vi "Key.vi"(4 "Comment (Create only)":string, 6 "Operation (Read or Create)":T1, 7 "Section":string, 8 "error in (no error)":errorcluster, 9 "Value":string, 10 "Key":string, 11 "Ini Path in":path) -> (0 "error out":errorcluster, 1 "Found?":bool, 2 "Value out":string, 3 "Ini Path out":path)   [LabVIEW 2021, in "Config.lvlib"]
uses:
  Config.lvlib
  TypeDefs/Operation.ctl
  TypeDefs/Action.ctl
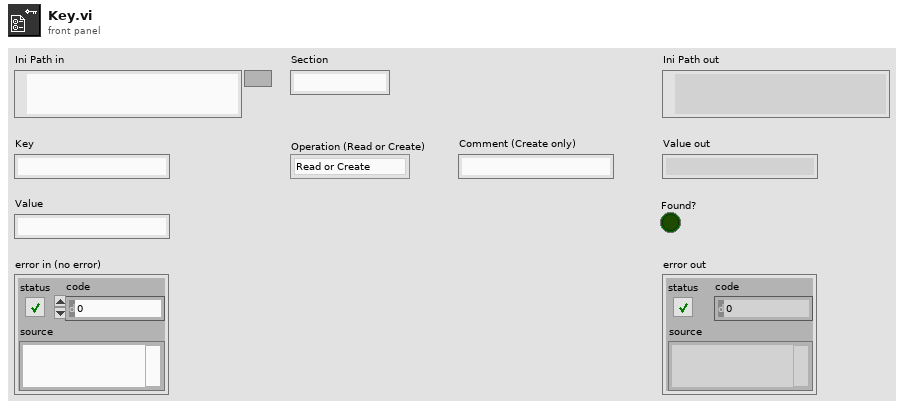
[diagram p1: front panel]
types:
  T1 = typedef "Config.lvlib/Operation.ctl" = enum8{"Read or Create", "Read", "Write"}
  T2 = typedef "Config.lvlib/Action.ctl" = enum8{"noop", "new", "read_or_create", "read", "write", "remove", "keys", "sections", "remove_section", "import", "export", "get", "set", "pop", "add", "list", "list_sections", "pop_section"}
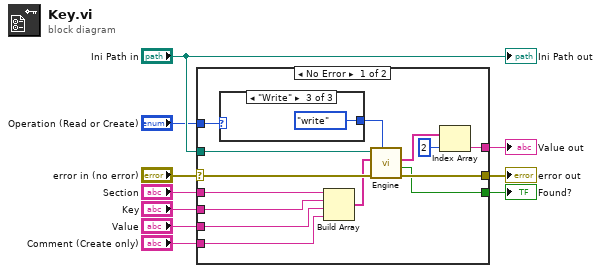
[diagram p0: block diagram]
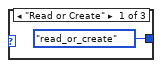
[diagram p2: hidden frame]
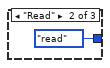
[diagram p3: hidden frame]
diagram:
  n1 = case shown="No Error" "error in (no error)" {
    selector: "error in (no error)" -> [w24 w29]
    tunnel: "Ini Path in" -> [w22 _]
    tunnel: [w21 w29] -> w8
    tunnel: "Section" -> [w20 _]
    tunnel: [w18 _] -> w6
    tunnel: "Key" -> [w17 _]
    tunnel: "Value" -> [w16 w28]
    tunnel: "Comment (Create only)" -> [w15 _]
    tunnel: "Operation (Read or Create)" -> [w14 _]
    tunnel: [w11 w28] -> w1
    frame No Error {
      n2 = case shown="\"Write\"" w14 {
        tunnel: [Action."read_or_create" ("Action") Action."read" ("Action") Action."write" ("Action")] -> w23
        frame "Read or Create" {
        }
        frame "Read" {
        }
        frame "Write" {
        }
      }
      n3 = Build Array(w20, w17, w16, w15) -> (w19:string[])
      n4 = call "Engine.vi"("Action"=w23, "error in (no error)"=w24, "skvc in"=w19, "INI Path in"=w22) -> ("error out"=w21:errorcluster, "Found?"=w18:bool, "skvc out"=w13:string[])  [unwired: 4 in, 1 out]
      n5 = Index Array(array=w13, index=2) -> (element=w11:string)
    }
    frame Error {
    }
  }
  "error out" <- w8
  "Found?" <- w6
  "Value out" <- w1
  "Ini Path out" <- "Ini Path in"
